vi "Write Pre-Addressed Observer Msgs.vi"(9 "Pre-Addressed Unsubscribe Msg":refnum<class "Unsubscribe Msg.lvclass">, 10 "Pre-Addressed Subscribe Msg":refnum<class "Subscribe Msg.lvclass">, 11 "IObserver In":refnum<class "IObserver.lvclass">) -> (3 "IObserver Out":refnum<class "IObserver.lvclass">)   [LabVIEW 2020, in "IObserver.lvlib" / "IObserver.lvclass"]
doc: "写入预先寻址的观察者消息"
uses:
  IObserver.lvclass
  IMediator/IMediator Messages/Subscribe Msg/Subscribe Msg.lvclass
  IMediator/IMediator Messages/Unsubscribe Msg/Unsubscribe Msg.lvclass
  IObserver.lvclass/IObserver.ctl
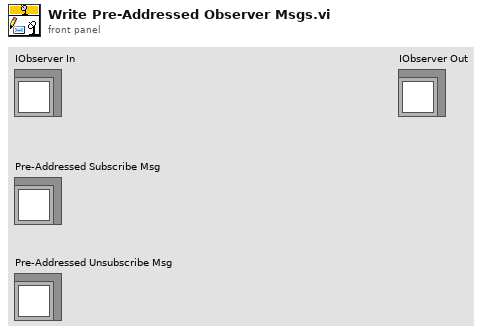
[diagram p1: front panel]
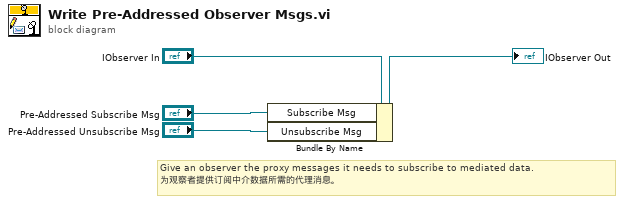
[diagram p0: block diagram]
diagram:
  # "Give an observer the proxy messages it needs to subscribe to mediated data.\n为观察者提供订阅中介数据所需的代理消息。"
  n1 = Bundle By Name(cluster="IObserver In", "Subscribe Msg"="Pre-Addressed Subscribe Msg", "Unsubscribe Msg"="Pre-Addressed Unsubscribe Msg") -> (→"IObserver Out":refnum<class "IObserver.lvclass">)
